vi "1. CalFocalFromKnowSquare.vi"() -> ()   [LabVIEW 2019]
panel:
  out "shiftDistance":dbl
  out "x-y":dbl
  out "newDistance":dbl[](array[numeric])
  out "right":sgl
  out "left":sgl
  out "element":T1
  out "f":dbl
  in  "RealDistance (cm)":dbl
  out "avg.length":dbl
  out "Image Out fgv 2":T2(plugin-control)
  out "Image Out fgv":T2(plugin-control)
  in  "stop":bool
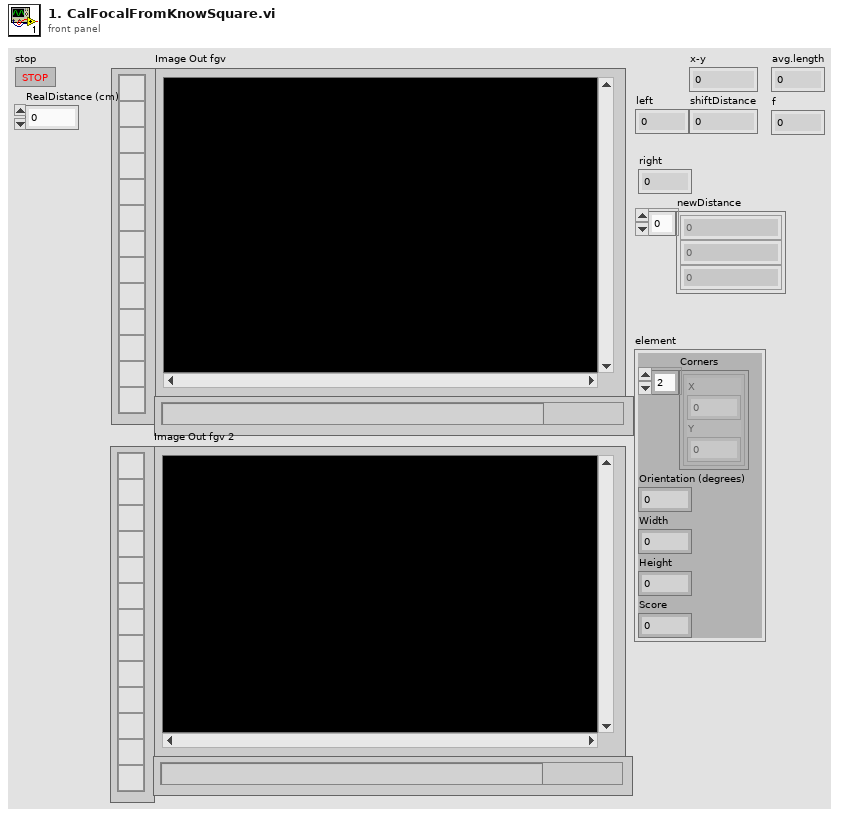
[diagram p1: front panel]
types:
  T1 = cluster{"Corners":cluster{"X":sgl, "Y":sgl}[], "Orientation (degrees)":dbl, "Width":dbl, "Height":dbl, "Score":dbl}
  T2 = typedef "IMAQ Image.ctl" = refnum<image>
  T3 = cluster{"Corners":cluster{"X":sgl, "Y":sgl}[], "Orientation (degrees)":dbl, "Width":dbl, "Height":dbl, "Score":dbl}[]
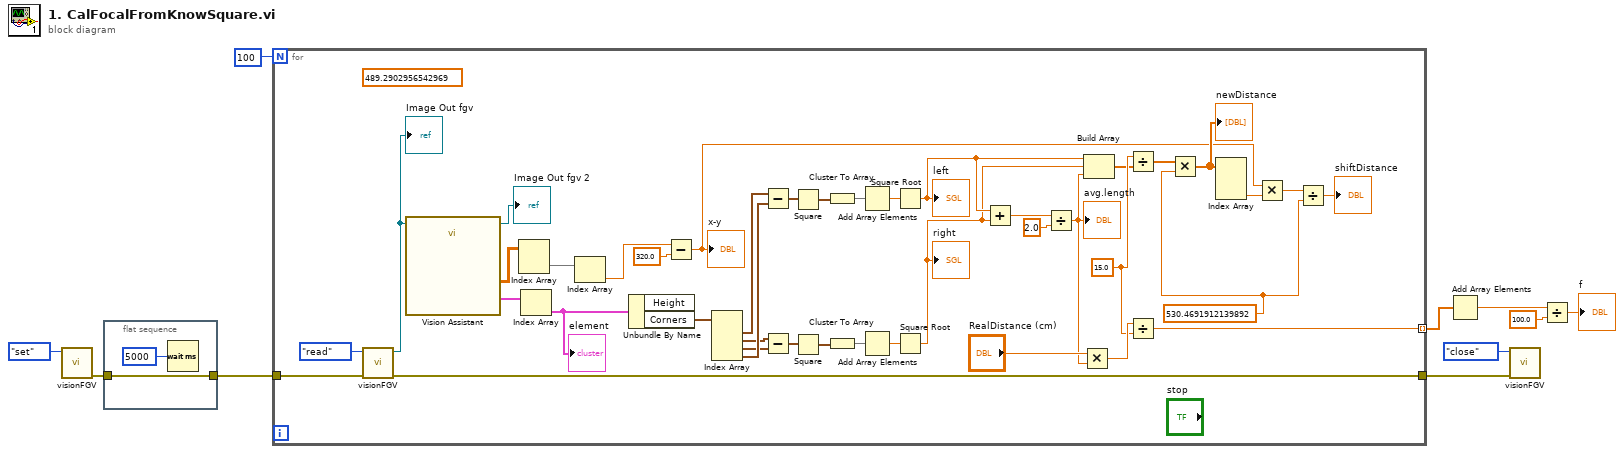
[diagram p0: block diagram]
diagram:
  n1 = call "visionFGV.vi"("Function"=enum16{"set", "read", "close"}."set") -> ("error out"=w1:errorcluster)  [unwired: 9 in, 1 out]
  n2 = flat-sequence {
    tunnel: [w12] -> w2
    tunnel: w1 -> [w12]
    frame #0 {
      n3 = Wait (ms)(milliseconds to wait=u32 5000) -> ()  [unwired: 1 out]
    }
  }
  n4 = for {
    N: 100 -> [_]
    tunnel: w2 -> [w53]
    tunnel: [w51] -> w8
    tunnel: [w24] -> w6 mode=indexing
    w13 = 530.4691912139892 ("f")
    (unwired) 489.2902956542969 ("f")
    w46 = 15.0 ("y")
    n5 = call "visionFGV.vi"("Error In"=w53, "Function"=enum16{"set", "read", "close"}."read") -> ("error out"=w51:errorcluster, "Image Out fgv"=w50:T2)  [unwired: 8 in]
    "Image Out fgv" <- w50
    n6 = call "Vision Assistant"("Image In"=w50) -> ("Image Out"=→"Image Out fgv 2":T2, "Rectangles (Shape Detection 1)"=w44:T3, "Particle Measurements (Pixels) (Particle Analysis 1)"=w23:dbl[][])  [unwired: 23 in, 1 out]
    n7 = Index Array(array=w23) -> (element=w22:dbl[])  [unwired: 2 in]
    n8 = Index Array(array=w44) -> (element=w43:T1)  [unwired: 1 in]
    "element" <- w43
    n9 = Index Array(array=w22) -> (element=w21:dbl)  [unwired: 1 in]
    n10 = Unbundle By Name(w43) -> ("Corners"=w42:cluster{"X":sgl, "Y":sgl}[])  [unwired: 1 out]
    n11 = Subtract(x=w21, y=320.0) -> (x-y=w17:dbl)
    "x-y" <- w17
    n12 = Index Array(array=w42) -> (element #1=w41:cluster{"X":sgl, "Y":sgl}, element #2=w39:cluster{"X":sgl, "Y":sgl}, element #3=w38:cluster{"X":sgl, "Y":sgl}, element #4=w40:cluster{"X":sgl, "Y":sgl})  [unwired: 4 in]
    n13 = Subtract(x=w41, y=w40) -> (x-y=w37:cluster{"X":sgl, "Y":sgl})
    n14 = Subtract(x=w39, y=w38) -> (x-y=w36:cluster{"X":sgl, "Y":sgl})
    n15 = Square(x=w37) -> (x^2=w35:cluster{"X":sgl, "Y":sgl})
    n16 = Square(x=w36) -> (x^2=w31:cluster{"X":sgl, "Y":sgl})
    n17 = Cluster To Array(cluster=w35) -> (array=w34:sgl[])
    n18 = Cluster To Array(cluster=w31) -> (array=w32:sgl[])
    n19 = Add Array Elements(numeric array=w34) -> (sum=w33:sgl)
    n20 = Add Array Elements(numeric array=w32) -> (sum=w30:sgl)
    n21 = Square Root(x=w33) -> (sqrt(x)=w28:sgl)
    "left" <- w28
    n22 = Square Root(x=w30) -> (sqrt(x)=w27:sgl)
    "right" <- w27
    n23 = Add(x=w28, y=w27) -> (x+y=w29:sgl)
    n24 = Divide(x=w29, y=sgl 2.0 ("x")) -> (x/y=w19:sgl)
    "avg.length" <- w19
    n25 = Multiply(x="RealDistance (cm)", y=w19) -> (x*y=w47:dbl)
    n26 = Build Array(w28, w27, w19) -> (w26:sgl[])
    n27 = Divide(x=w46, y=w26) -> (x/y=w45:dbl[])
    n28 = Divide(x=w47, y=w46) -> (x/y=w24:dbl)
    n29 = Multiply(x=w45, y=w13) -> (x*y=w18:dbl[])
    "newDistance" <- w18
    n30 = Index Array(array=w18) -> (element #3=w16:dbl)  [unwired: 3 in, 2 out]
    n31 = Multiply(x=w17, y=w16) -> (x*y=w15:dbl)
    n32 = Divide(x=w15, y=w13) -> (x/y=→"shiftDistance":dbl)
  }
  n33 = Add Array Elements(numeric array=w6) -> (sum=w5:dbl)
  n34 = call "visionFGV.vi"("Error In"=w8, "Function"=enum16{"set", "read", "close"}."close") -> ()  [unwired: 8 in, 2 out]
  n35 = Divide(x=w5, y=100.0) -> (x/y=→"f":dbl)
